vi "TriggerTime.vi"(8 "error in (no error)":errorcluster, 9 "TriggerTime":dbl, 10 "ModuleID":i32) -> (0 "error out":errorcluster)   [LabVIEW 2014, in "SyncModule.lvlib"]
uses:
  SyncModule.lvlib
  clEventType.ctl
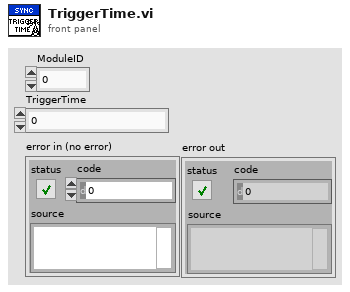
[diagram p1: front panel]
types:
  T1 = typedef "SyncModule.lvlib/clEventType.ctl" = cluster{"ModuleID":i32, "Data":variant}
  T2 = typedef "SyncModule.lvlib/clBroadcastEvents.ctl" = cluster{"DidInit":refnum<user-event>, "StatusUpdate":refnum<user-event>, "ErrorReport":refnum<user-event>, "DidStop":refnum<user-event>, "PathToINI":refnum<user-event>, "TriggerTime":refnum<user-event>}
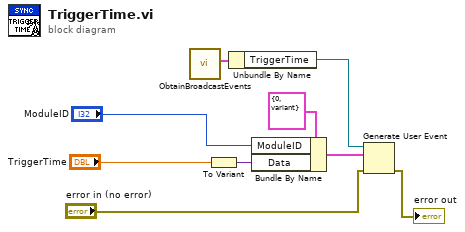
[diagram p0: block diagram]
diagram:
  n1 = call "ObtainBroadcastEvents.vi"() -> ("clBroadcastEvents"=w9:T2)  [unwired: 10 in, 1 out]
  n2 = To Variant(anything="TriggerTime") -> (Variant=w6:variant)
  n3 = Unbundle By Name(w9) -> ("TriggerTime"=w8:refnum<user-event>)
  n4 = Bundle By Name(cluster=T1 {"ModuleID"=0, "Data"=variant} ("clBroadcast"), "ModuleID"="ModuleID", "Data"=w6) -> (w5:T1)
  n5 = Generate User Event(user event=w8, event data cluster=w5, error in="error in (no error)") -> (error out=→"error out":errorcluster)  [unwired: 1 in, 1 out]
